vi "Controller.vi"(8 "error in (no error)":errorcluster) -> (0 "error out":errorcluster)   [LabVIEW 2021]
uses:
  QueueEnum.ctl
  ControlerStatus.ctl
  ModelQueueCluster.ctl
  ToModelSourceEnum.ctl
  FromTCPCluster.ctl
  ToModelFromTCPMessage.ctl
  FormControllerToMOdelCluster.ctl
  ToModelFromControllerEnum.ctl
  ViewUpdateEnum.ctl
  TCPQueueData.ctl
  TCPModuleState.ctl
  ToViewQueueData.ctl
  ToLoggerQueueCluster.ctl
  LoggerEnum.ctl
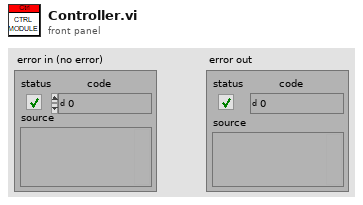
[diagram p1: front panel]
types:
  T1 = typedef "ControlerStatus.ctl" = cluster{"ConnectionState":bool, "Log Status":bool}
  T2 = enum32{"Invalid", "Standard", "Closed", "Hidden", "Minimized", "Maximized"}
  T3 = typedef "QueueEnum.ctl" = enum16{"Obtain Queue", "Get Queue Ref", "Flush Queue", "Release Queue"}
  T4 = typedef "ToModelFromControllerEnum.ctl" = enum16{"StopLogging", "StartLogging", "SlideChange", "SendMessage", "Exit", "Disconnect", "Connect"}
  T5 = typedef "ToModelSourceEnum.ctl" = enum16{"TCP", "Controller"}
  T6 = typedef "ModelQueueCluster.ctl" = cluster{"Source":T5, "FromTCPCluster":T7, "FromControllerCluster":T9}
  T7 = typedef "FromTCPCluster.ctl" = cluster{"Message":T8, "Data":string, "StatusOK?":bool}
  T8 = typedef "ToModelFromTCPMessage.ctl" = enum16{"Exit", "DataWritten", "DataReceived", "Timeout", "UnableToConnect", "Disconnected", "Connected"}
  T9 = typedef "FormControllerToMOdelCluster.ctl" = cluster{"Command":T4, "IP Address":string, "Remote Port":u16, "Data":string, "TCP/COM":bool, "VISA resource name":refnum<visa-resource-name>}
  T10 = typedef "LoggerEnum.ctl" = enum16{"StartLogging", "StopLogging", "ReadData", "SendData", "WriteData", "Exit"}
  T11 = typedef "ToLoggerQueueCluster.ctl" = cluster{"Command":T10, "Data":dbl[][], "Path":path}
  T12 = typedef "ToViewQueueData.ctl" = cluster{"DataToUpdate":T13, "ConnectionStatus":bool, "GraphData":dbl[][], "Message":string, "TCP/COM":bool}
  T13 = typedef "ViewUpdateEnum.ctl" = enum16{"Init", "OneButtonMessage", "Exit", "UpdateButtonsEnabled", "UpdateGraph", "UpdateConnectionStatus", "UpdateCOMList"}
  T14 = typedef "TCPModuleState.ctl" = enum16{"Init", "Connect", "Read", "Write", "Disconnect", "ErrorHandler", "Exit"}
  T15 = typedef "TCPQueueData.ctl" = cluster{"Command":T14, "address":string, "remote port":u16, "Data":string}
  T16 = typedef "ToControllerQueueCluster.ctl" = cluster{"Message":T17, "Remote IP":string, "Remote Port":u16, "Data":string, "TCP/COM":bool, "COM Port":string}
  T17 = typedef "ToControllerEnum.ctl" = enum16{"Info_Disconnected", "Info_Connected", "Exit", "Disconnect", "Connect", "SendMessage", "Slide", "ShowDataFromLog", "Start_Saving_Logs", "Stop_Saving_Logs"}
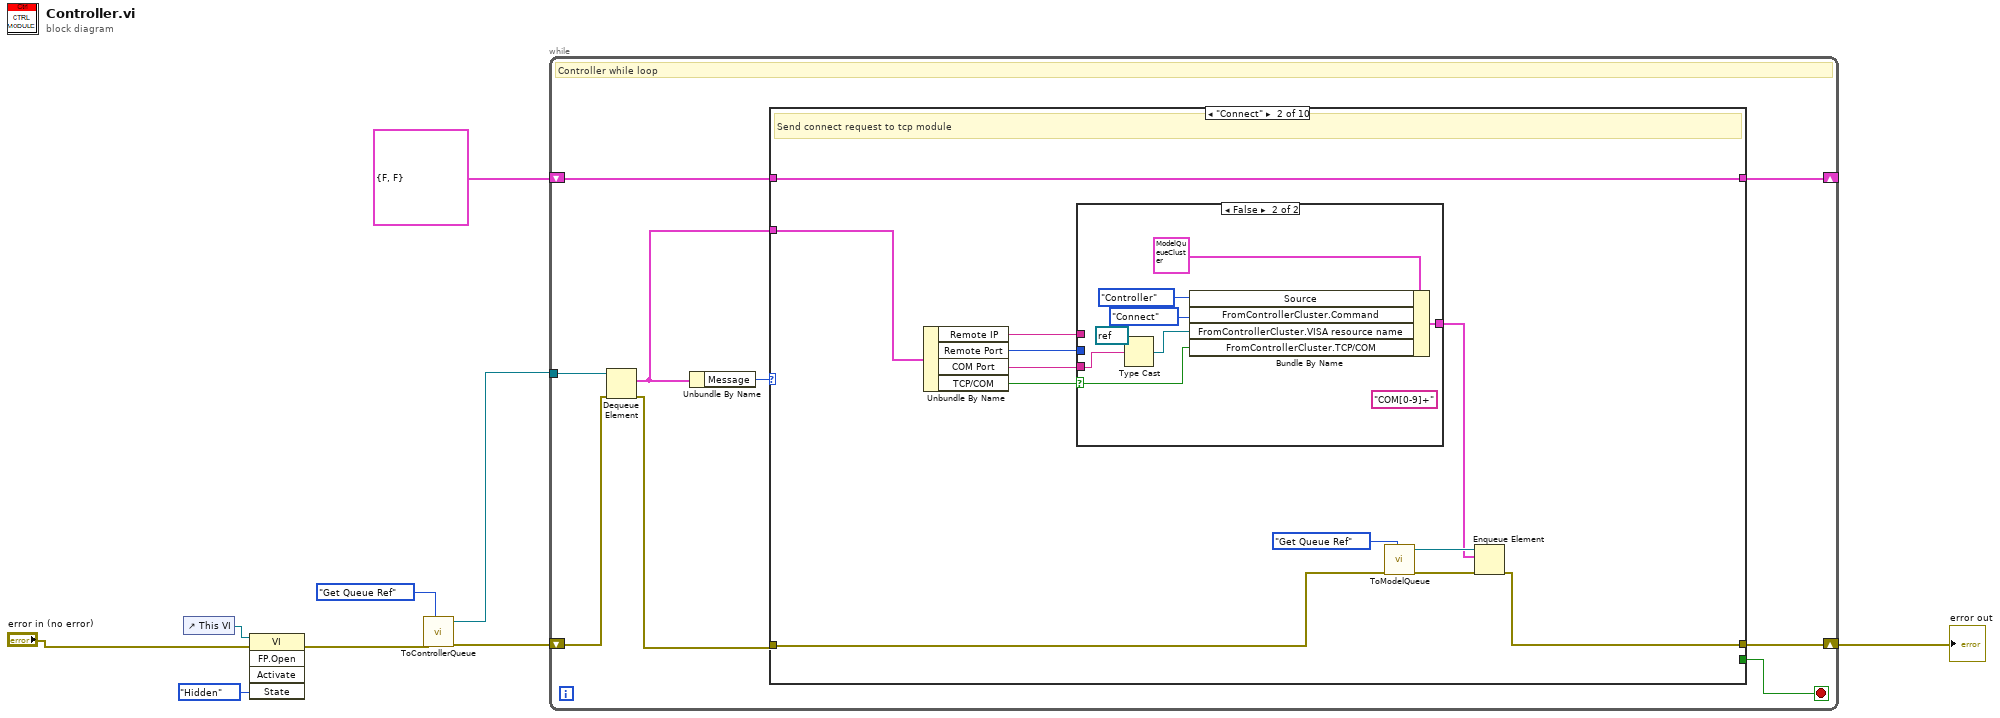
[diagram p0: block diagram]
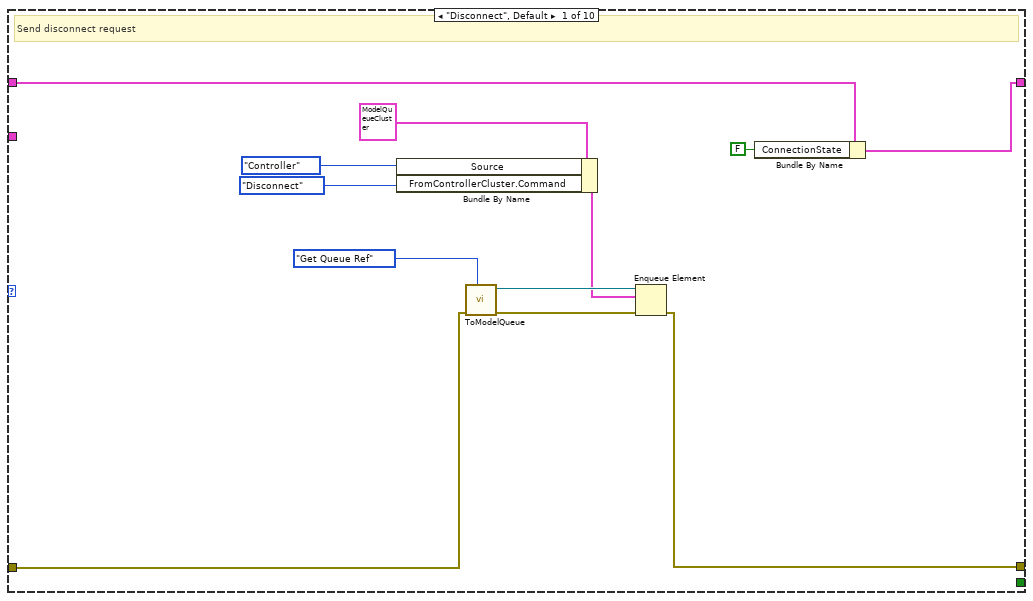
[diagram p2: hidden frame]
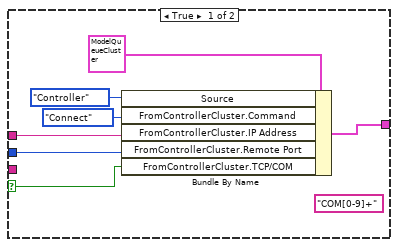
[diagram p3: hidden frame]
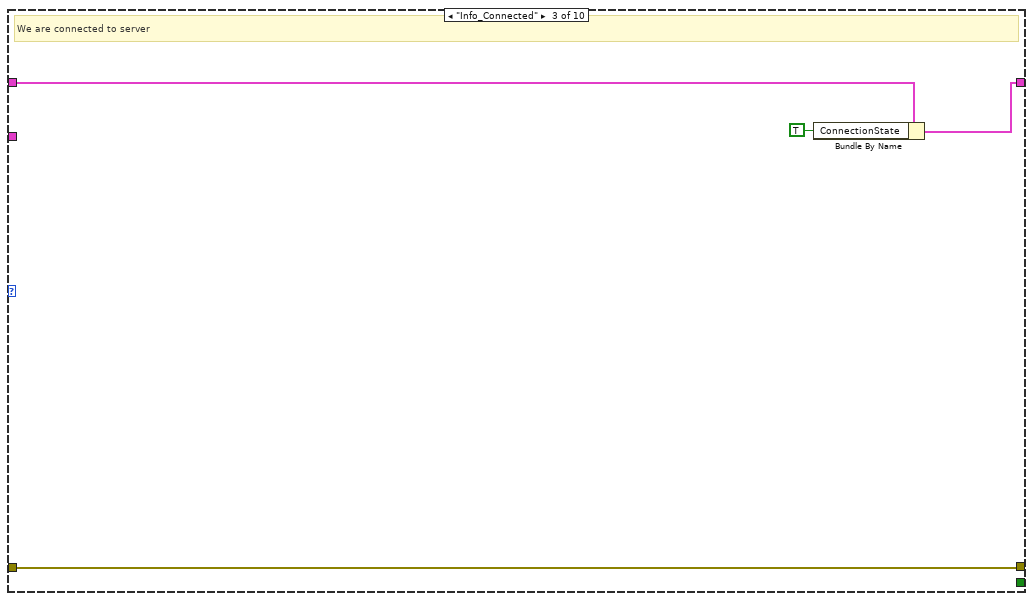
[diagram p4: hidden frame]
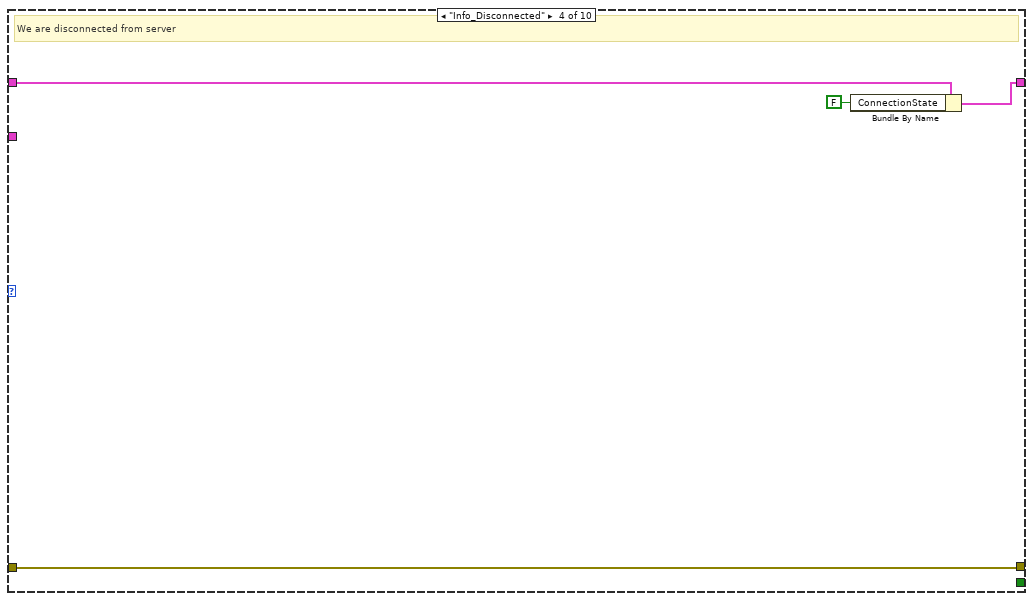
[diagram p5: hidden frame]
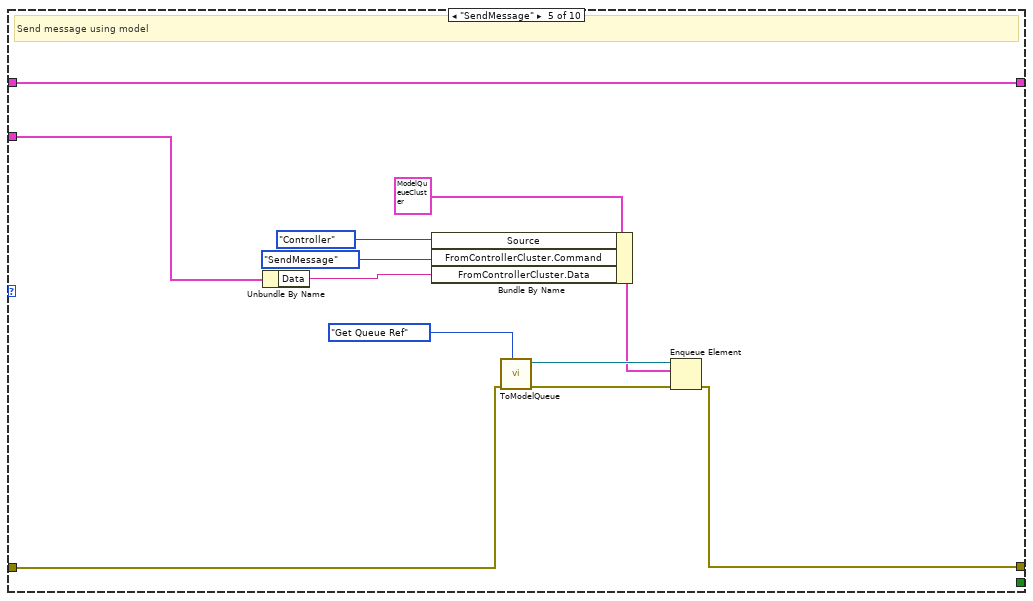
[diagram p6: hidden frame]
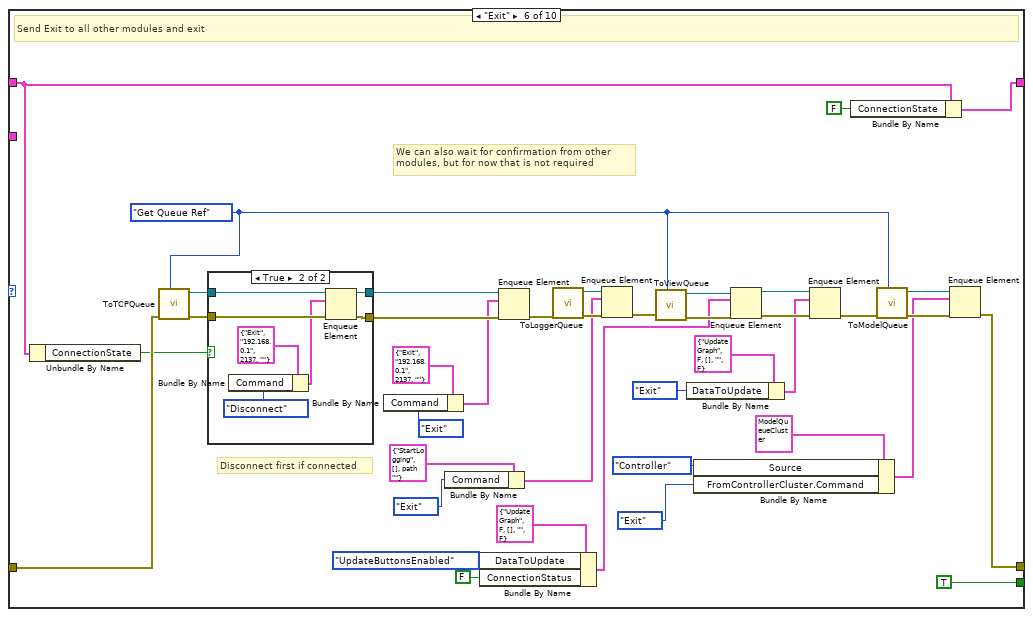
[diagram p7: hidden frame]
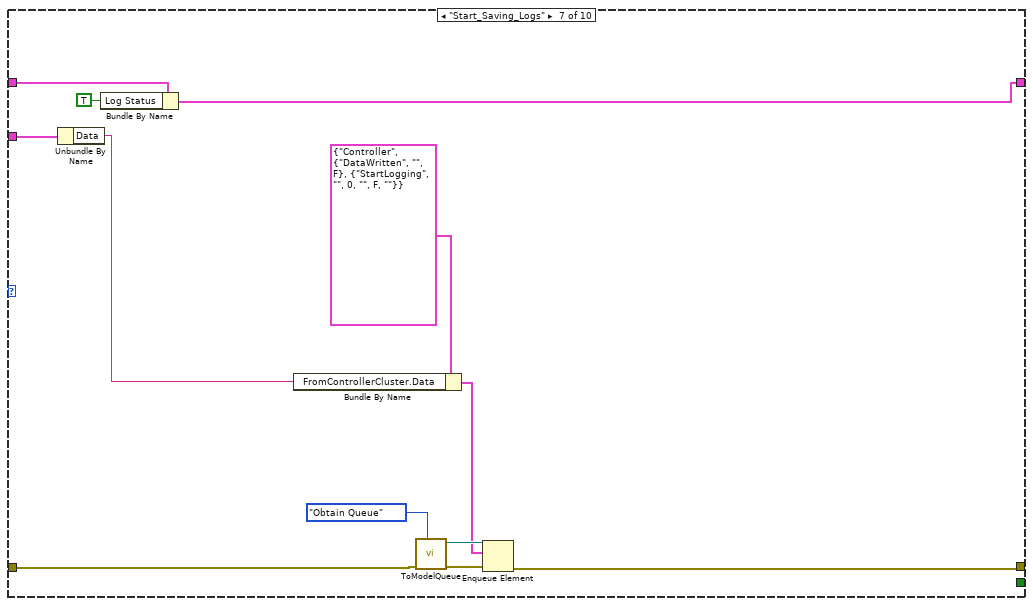
[diagram p9: hidden frame]
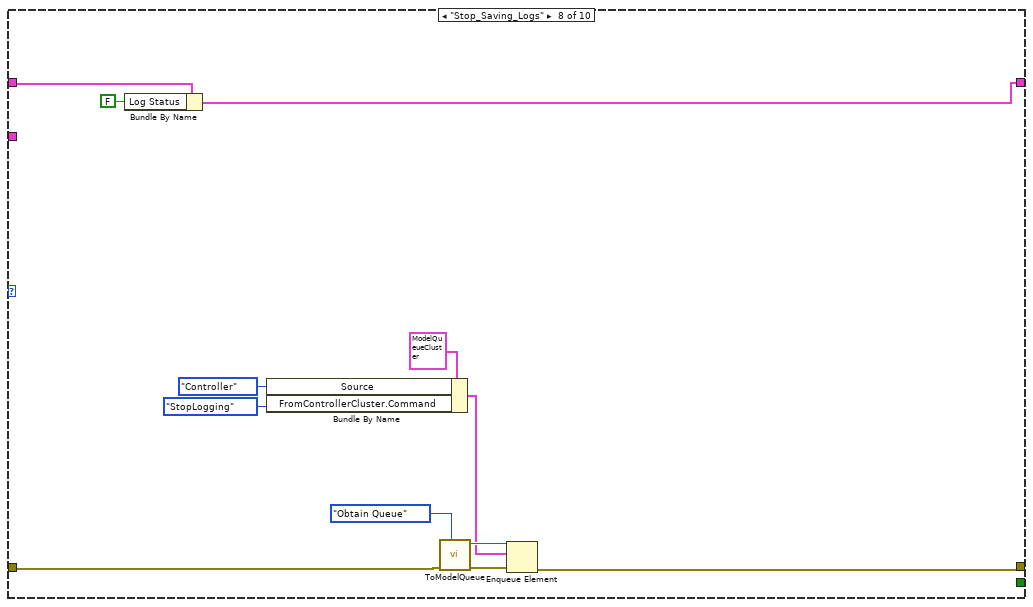
[diagram p10: hidden frame]
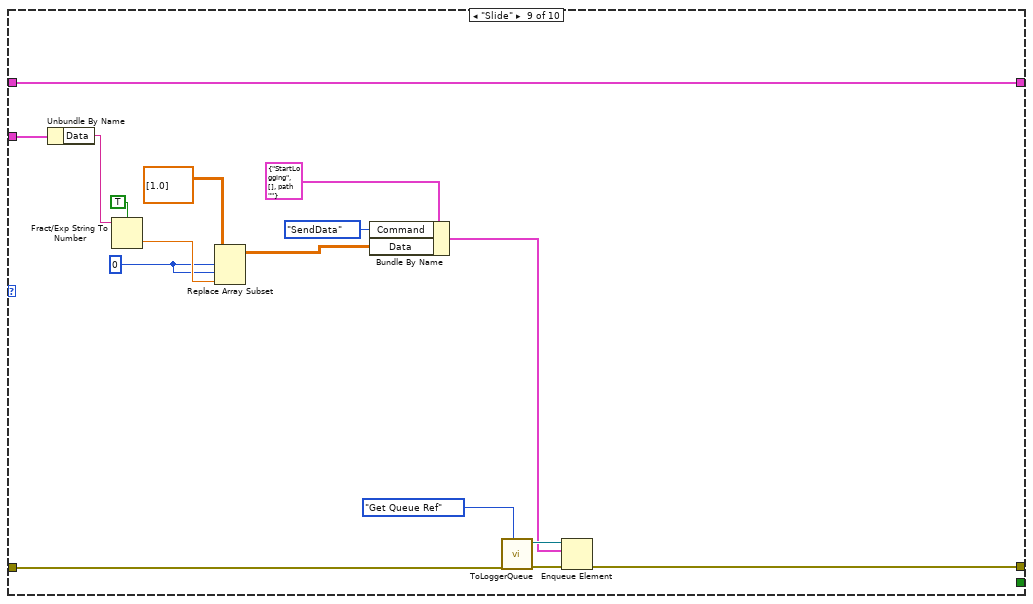
[diagram p11: hidden frame]
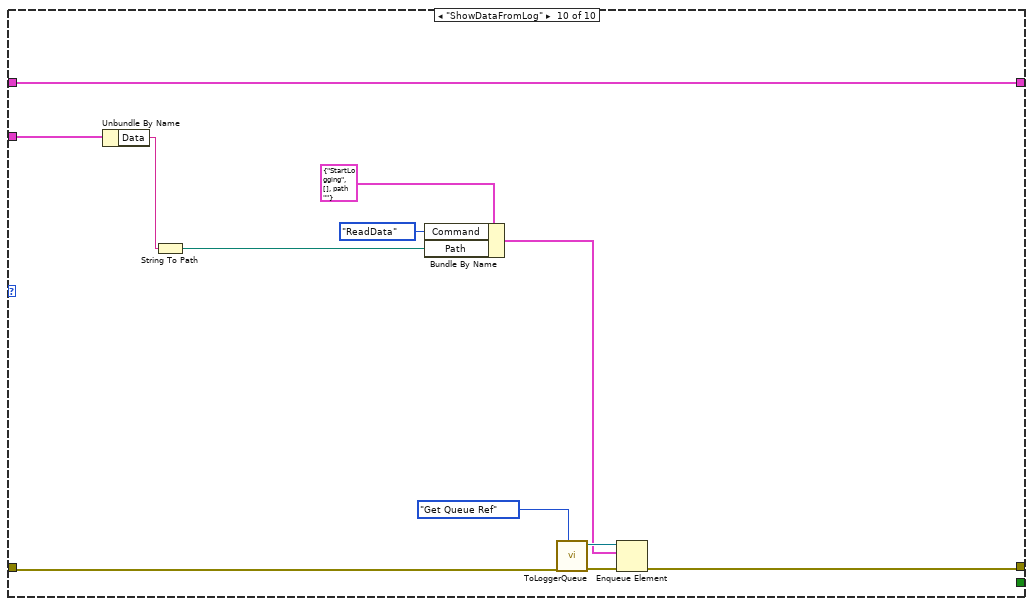
[diagram p12: hidden frame]
diagram:
  n1 = control-ref of="This VI"() -> (w5:refnum<vi>)
  n2 = invoke class="VI" method="FP.Open"(reference=w5, error in="error in (no error)", "State"=T2."Hidden") -> (error out=w2:errorcluster)  [unwired: 2 in, 4 out]
  n3 = call "ToControllerQueue.vi"("Enum"=QueueEnum."Get Queue Ref", "error in (no error)"=w2) -> ("error out"=w9:errorcluster, "queue out"=w7:refnum<queue>)  [unwired: 8 in]
  n4 = while {
    tunnel: w7 -> [w18]
    shift-right: [w13] -> w6
    shift-left: w9 -> [w17]
    shift-right: [w10] -> _
    shift-left: T1 {"ConnectionState"=FALSE, "Log Status"=FALSE} -> [w11]
    stop <- w12 stop-if-true
    # "Controller while loop"
    n5 = Dequeue Element(queue=w18, error in (no error)=w17) -> (element=w15:T16, error out=w14:errorcluster)  [unwired: 1 in, 2 out]
    n6 = Unbundle By Name(w15) -> ("Message"=w16:T17)
    n7 = case shown="\"Connect\"" w16 {
      tunnel: w15 -> [_ w42 _ _ w77 _ w130 _ w161 w170]
      tunnel: w14 -> [w27 w37 w61 w65 w69 w102 w138 w144 w165 w172]
      tunnel: [w26 w36 w61 w65 w68 w108 w131 w143 w162 w171] -> w13
      tunnel: [_ _ _ _ _ TRUE _ _ _ _] -> w12
      tunnel: w11 -> [w21 w33 w60 w64 w66 w86 w136 w146 w166 w167]
      tunnel: [w19 w33 w59 w63 w66 w88 w134 w145 w166 w167] -> w10
      frame "Disconnect", Default {
        # "Send disconnect request"
        n8 = Bundle By Name(cluster=T6 {"Source"=enum."Controller", "FromTCPCluster"={"Message"=enum."DataWritten", "Data"="", "StatusOK?"=FALSE}, "FromControllerCluster"={"Command"=enum."Disconnect", "IP Address"="192.168.0.1", "Remote Port"=2137, "Data"="", "TCP/COM"=FALSE, "VISA resource name"=""}} ("element"), "Source"=ToModelSourceEnum."Controller", "FromControllerCluster.Command"=ToModelFromControllerEnum."Disconnect" ("FromControllerCluster.Enum")) -> (w22:T6)
        n9 = call "ToModelQueue.vi"("Enum"=QueueEnum."Get Queue Ref", "error in (no error)"=w27) -> ("error out"=w29:errorcluster, "queue out"=w28:refnum<queue>)  [unwired: 8 in]
        n10 = Enqueue Element(queue=w28, element=w22, error in (no error)=w29) -> (error out=w26:errorcluster)  [unwired: 1 in, 2 out]
        n11 = Bundle By Name(cluster=w21, "ConnectionState"=FALSE) -> (w19:T1)
      }
      frame "Connect" {
        # "Send connect request to tcp module"
        n12 = Unbundle By Name(w42) -> ("Remote IP"=w35:string, "Remote Port"=w34:u16, "COM Port"=w31:string, "TCP/COM"=w32:bool)
        n13 = case shown="False" w32 {
          selector: w32 -> [w43 w50]
          tunnel: [w46 w54] -> w38
          tunnel: w35 -> [w45 _]
          tunnel: w34 -> [w44 _]
          tunnel: w31 -> [_ w53]
          frame True {
            (unwired) "COM[0-9]+" ("regular expression")
            n14 = Bundle By Name(cluster=T6 {"Source"=enum."Controller", "FromTCPCluster"={"Message"=enum."DataWritten", "Data"="", "StatusOK?"=FALSE}, "FromControllerCluster"={"Command"=enum."Disconnect", "IP Address"="192.168.0.1", "Remote Port"=2137, "Data"="", "TCP/COM"=FALSE, "VISA resource name"=""}} ("element"), "Source"=ToModelSourceEnum."Controller", "FromControllerCluster.Command"=ToModelFromControllerEnum."Connect" ("FromControllerCluster.Enum"), "FromControllerCluster.IP Address"=w45, "FromControllerCluster.Remote Port"=w44, "FromControllerCluster.TCP/COM"=w43) -> (w46:T6)
          }
          frame False {
            (unwired) "COM[0-9]+" ("regular expression")
            n15 = Type Cast(type=refnum<visa-resource-name> refnum ("VISA resource name"), x=w53) -> (*(type *) &x=w51:refnum<visa-resource-name>)
            n16 = Bundle By Name(cluster=T6 {"Source"=enum."Controller", "FromTCPCluster"={"Message"=enum."DataWritten", "Data"="", "StatusOK?"=FALSE}, "FromControllerCluster"={"Command"=enum."Disconnect", "IP Address"="192.168.0.1", "Remote Port"=2137, "Data"="", "TCP/COM"=FALSE, "VISA resource name"=""}} ("element"), "Source"=ToModelSourceEnum."Controller", "FromControllerCluster.Command"=ToModelFromControllerEnum."Connect" ("FromControllerCluster.Enum"), "FromControllerCluster.VISA resource name"=w51, "FromControllerCluster.TCP/COM"=w50) -> (w54:T6)
          }
        }
        n17 = call "ToModelQueue.vi"("Enum"=QueueEnum."Get Queue Ref", "error in (no error)"=w37) -> ("error out"=w40:errorcluster, "queue out"=w39:refnum<queue>)  [unwired: 8 in]
        n18 = Enqueue Element(queue=w39, element=w38, error in (no error)=w40) -> (error out=w36:errorcluster)  [unwired: 1 in, 2 out]
      }
      frame "Info_Connected" {
        # "We are connected to server"
        n19 = Bundle By Name(cluster=w60, "ConnectionState"=TRUE) -> (w59:T1)
      }
      frame "Info_Disconnected" {
        # "We are disconnected from server"
        n20 = Bundle By Name(cluster=w64, "ConnectionState"=FALSE) -> (w63:T1)
      }
      frame "SendMessage" {
        # "Send message using model"
        n21 = Unbundle By Name(w77) -> ("Data"=w67:string)
        n22 = Bundle By Name(cluster=T6 {"Source"=enum."Controller", "FromTCPCluster"={"Message"=enum."DataWritten", "Data"="", "StatusOK?"=FALSE}, "FromControllerCluster"={"Command"=enum."Disconnect", "IP Address"="192.168.0.1", "Remote Port"=2137, "Data"="", "TCP/COM"=FALSE, "VISA resource name"=""}} ("element"), "Source"=ToModelSourceEnum."Controller", "FromControllerCluster.Command"=ToModelFromControllerEnum."SendMessage" ("FromControllerCluster.Enum"), "FromControllerCluster.Data"=w67) -> (w70:T6)
        n23 = call "ToModelQueue.vi"("Enum"=QueueEnum."Get Queue Ref", "error in (no error)"=w69) -> ("error out"=w75:errorcluster, "queue out"=w74:refnum<queue>)  [unwired: 8 in]
        n24 = Enqueue Element(queue=w74, element=w70, error in (no error)=w75) -> (error out=w68:errorcluster)  [unwired: 1 in, 2 out]
      }
      frame "Exit" {
        w110 = QueueEnum."Get Queue Ref"
        # "Disconnect first if connected"
        # "We can also wait for confirmation from other\nmodules, but for now that is not required"
        # "Send Exit to all other modules and exit"
        n25 = Unbundle By Name(w86) -> ("ConnectionState"=w85:bool)
        n26 = call "ToTCPQueue.vi"("Enum"=w110, "error in (no error)"=w102) -> ("error out"=w116:errorcluster, "queue out"=w115:refnum<queue>)  [unwired: 8 in]
        n27 = case shown="True" w85 {
          tunnel: w116 -> [w119 w126]
          tunnel: [w119 w125] -> w101
          tunnel: w115 -> [w118 w124]
          tunnel: [w118 w120] -> w100
          frame False {
          }
          frame True {
            n28 = Bundle By Name(cluster=T15 {"Command"=enum."Exit", "address"="192.168.0.1", "remote port"=2137, "Data"=""} ("element"), "Command"=TCPModuleState."Disconnect") -> (w122:T15)
            n29 = Enqueue Element(queue=w124, element=w122, error in (no error)=w126) -> (queue out=w120:refnum<queue>, error out=w125:errorcluster)  [unwired: 1 in, 1 out]
          }
        }
        n30 = Bundle By Name(cluster=T15 {"Command"=enum."Exit", "address"="192.168.0.1", "remote port"=2137, "Data"=""} ("element"), "Command"=TCPModuleState."Exit") -> (w97:T15)
        n31 = Bundle By Name(cluster=T11 {"Command"=enum."StartLogging", "Data"=[], "Path"=path ""} ("element"), "Command"=LoggerEnum."Exit") -> (w79:T11)
        n32 = Bundle By Name(cluster=T12 {"DataToUpdate"=enum."UpdateGraph", "ConnectionStatus"=FALSE, "GraphData"=[], "Message"="", "TCP/COM"=FALSE} ("element"), "DataToUpdate"=ViewUpdateEnum."UpdateButtonsEnabled", "ConnectionStatus"=FALSE) -> (w90:T12)
        n33 = Enqueue Element(queue=w100, element=w97, error in (no error)=w101) -> (error out=w84:errorcluster)  [unwired: 1 in, 2 out]
        n34 = call "ToLoggerQueue.vi"("error in (no error)"=w84) -> ("error out"=w83:errorcluster, "queue out"=w81:refnum<queue>)  [unwired: 9 in]
        n35 = Enqueue Element(queue=w81, element=w79, error in (no error)=w83) -> (error out=w82:errorcluster)  [unwired: 1 in, 2 out]
        n36 = call "ToViewQueue.vi"("Enum"=w110, "error in (no error)"=w82) -> ("error out"=w114:errorcluster, "queue out"=w113:refnum<queue>)  [unwired: 8 in]
        n37 = Bundle By Name(cluster=T12 {"DataToUpdate"=enum."UpdateGraph", "ConnectionStatus"=FALSE, "GraphData"=[], "Message"="", "TCP/COM"=FALSE} ("element"), "DataToUpdate"=ViewUpdateEnum."Exit") -> (w94:T12)
        n38 = Bundle By Name(cluster=T6 {"Source"=enum."Controller", "FromTCPCluster"={"Message"=enum."DataWritten", "Data"="", "StatusOK?"=FALSE}, "FromControllerCluster"={"Command"=enum."Disconnect", "IP Address"="192.168.0.1", "Remote Port"=2137, "Data"="", "TCP/COM"=FALSE, "VISA resource name"=""}} ("element"), "Source"=ToModelSourceEnum."Controller", "FromControllerCluster.Command"=ToModelFromControllerEnum."Exit" ("FromControllerCluster.Enum")) -> (w103:T6)
        n39 = Enqueue Element(queue=w113, element=w90, error in (no error)=w114) -> (queue out=w89:refnum<queue>, error out=w96:errorcluster)  [unwired: 1 in, 1 out]
        n40 = Enqueue Element(queue=w89, element=w94, error in (no error)=w96) -> (error out=w95:errorcluster)  [unwired: 1 in, 2 out]
        n41 = Bundle By Name(cluster=w86, "ConnectionState"=FALSE) -> (w88:T1)
        n42 = call "ToModelQueue.vi"("Enum"=w110, "error in (no error)"=w95) -> ("error out"=w109:errorcluster, "queue out"=w107:refnum<queue>)  [unwired: 8 in]
        n43 = Enqueue Element(queue=w107, element=w103, error in (no error)=w109) -> (error out=w108:errorcluster)  [unwired: 1 in, 2 out]
      }
      frame "Start_Saving_Logs" {
        n44 = Unbundle By Name(w130) -> ("Data"=w129:string)
        n45 = Bundle By Name(cluster=w136, "Log Status"=TRUE) -> (w134:T1)
        n46 = Bundle By Name(cluster=T6 {"Source"=enum."Controller", "FromTCPCluster"={"Message"=enum."DataWritten", "Data"="", "StatusOK?"=FALSE}, "FromControllerCluster"={"Command"=enum."StartLogging", "IP Address"="", "Remote Port"=0, "Data"="", "TCP/COM"=FALSE, "VISA resource name"=""}} ("element"), "FromControllerCluster.Data"=w129) -> (w128:T6)
        n47 = call "ToModelQueue.vi"("Enum"=QueueEnum."Obtain Queue", "error in (no error)"=w138) -> ("error out"=w132:errorcluster, "queue out"=w133:refnum<queue>)  [unwired: 8 in]
        n48 = Enqueue Element(queue=w133, element=w128, error in (no error)=w132) -> (error out=w131:errorcluster)  [unwired: 1 in, 2 out]
      }
      frame "Stop_Saving_Logs" {
        n49 = Bundle By Name(cluster=w146, "Log Status"=FALSE) -> (w145:T1)
        n50 = Bundle By Name(cluster=T6 {"Source"=enum."Controller", "FromTCPCluster"={"Message"=enum."DataWritten", "Data"="", "StatusOK?"=FALSE}, "FromControllerCluster"={"Command"=enum."StopLogging", "IP Address"="", "Remote Port"=0, "Data"="", "TCP/COM"=FALSE, "VISA resource name"=""}} ("element"), "Source"=ToModelSourceEnum."Controller", "FromControllerCluster.Command"=ToModelFromControllerEnum."StopLogging") -> (w139:T6)
        n51 = call "ToModelQueue.vi"("Enum"=QueueEnum."Obtain Queue", "error in (no error)"=w144) -> ("error out"=w147:errorcluster, "queue out"=w148:refnum<queue>)  [unwired: 8 in]
        n52 = Enqueue Element(queue=w148, element=w139, error in (no error)=w147) -> (error out=w143:errorcluster)  [unwired: 1 in, 2 out]
      }
      frame "Slide" {
        w152 = 0 ("index (row)")
        n53 = Unbundle By Name(w161) -> ("Data"=w157:string)
        n54 = Fract/Exp String To Number(use system decimal point (T)=TRUE, string=w157) -> (number=w153:dbl)  [unwired: 2 in, 1 out]
        n55 = Replace Array Subset(array=dbl[][] [[1.0]], new element=w153, index (row)=w152, index (col)=w152) -> (w155:dbl[][])
        n56 = Bundle By Name(cluster=T11 {"Command"=enum."StartLogging", "Data"=[], "Path"=path ""} ("element"), "Command"=LoggerEnum."SendData", "Data"=w155) -> (w151:T11)
        n57 = call "ToLoggerQueue.vi"("Enum"=QueueEnum."Get Queue Ref", "error in (no error)"=w165) -> ("error out"=w163:errorcluster, "queue out"=w164:refnum<queue>)  [unwired: 8 in]
        n58 = Enqueue Element(queue=w164, element=w151, error in (no error)=w163) -> (error out=w162:errorcluster)  [unwired: 1 in, 2 out]
      }
      frame "ShowDataFromLog" {
        n59 = Unbundle By Name(w170) -> ("Data"=w169:string)
        n60 = String To Path(string=w169) -> (path=w168:path)
        n61 = Bundle By Name(cluster=T11 {"Command"=enum."StartLogging", "Data"=[], "Path"=path ""} ("element"), "Command"=LoggerEnum."ReadData", "Path"=w168) -> (w173:T11)
        n62 = call "ToLoggerQueue.vi"("Enum"=QueueEnum."Get Queue Ref", "error in (no error)"=w172) -> ("error out"=w177:errorcluster, "queue out"=w178:refnum<queue>)  [unwired: 8 in]
        n63 = Enqueue Element(queue=w178, element=w173, error in (no error)=w177) -> (error out=w171:errorcluster)  [unwired: 1 in, 2 out]
      }
    }
  }
  "error out" <- w6
